vi "read_params.vi"(8 "error in (no error)":errorcluster, 11 "MLPRegressor in":refnum<class "MLPRegressor.lvclass">) -> (0 "error out":errorcluster, 2 "params":T1={"hidden_layer_sizes"=[100.0], "activation"="relu", "solver"="adam", "alpha"=0.0001, "batch_size"={"batch_size_type"="auto", "batch_size_int"=32.0}, "learning_rate"="constant", "learning_rate_init"=0.001, "power_t"=0.5, "max_iter"=200.0, "shuffle"=TRUE, "random_state"=0.0, "tol"=0.0001, "verbose"=FALSE, "warm_start"=FALSE, "momentum"=0.9, "nesterovs_momentum"=FALSE, "early_stopping"=FALSE, "validation_fraction"=0.1, "beta_1"=0.999, "beta_2"=0.999, "epsilon"=1e-08, "n_iter_no_change"=10.0, "max_fun"=15000.0}, 3 "MLPRegressor out":refnum<class "MLPRegressor.lvclass">)   [LabVIEW 2020, in "MLPRegressor.lvclass"]
uses:
  MLPRegressor.lvclass
  Controls/mlp_regressor_params.ctl
  MLPRegressor.lvclass/MLPRegressor.ctl
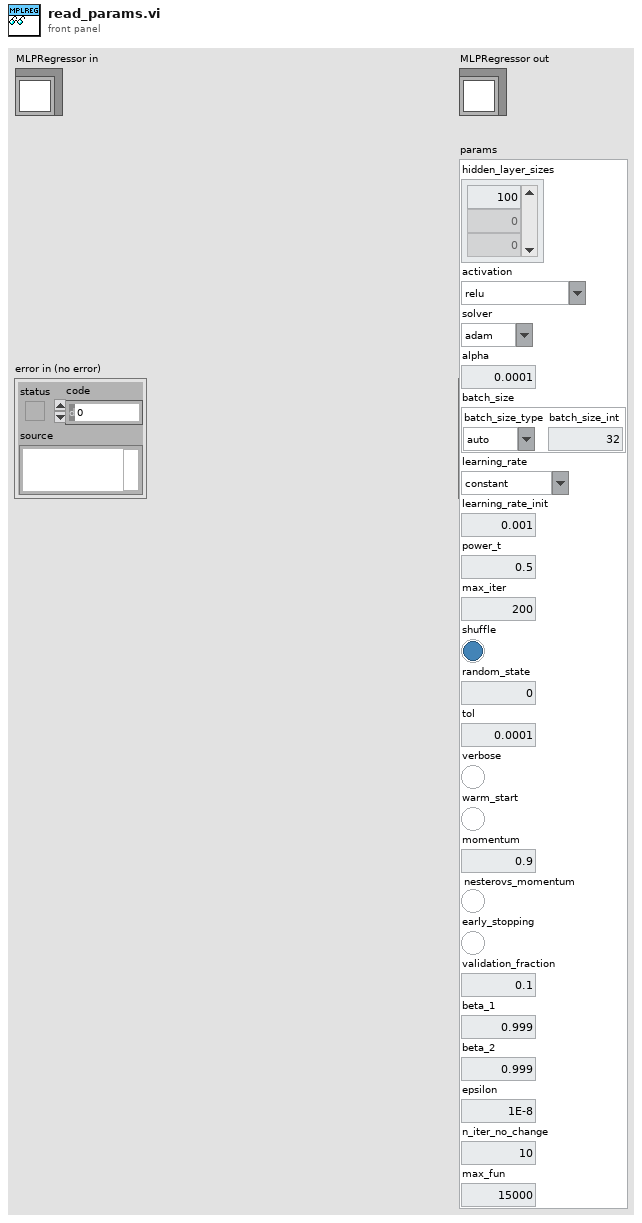
[diagram p1: front panel]
types:
  T1 = typedef "mlp_regressor_params.ctl" = cluster{"hidden_layer_sizes":dbl[], "activation":string, "solver":string, "alpha":dbl, "batch_size":cluster{"batch_size_type":string, "batch_size_int":dbl}, "learning_rate":string, "learning_rate_init":dbl, "power_t":dbl, "max_iter":dbl, "shuffle":bool, "random_state":dbl, "tol":dbl, "verbose":bool, "warm_start":bool, "momentum":dbl, "nesterovs_momentum":bool, "early_stopping":bool, "validation_fraction":dbl, "beta_1":dbl, "beta_2":dbl, "epsilon":dbl, "n_iter_no_change":dbl, "max_fun":dbl}
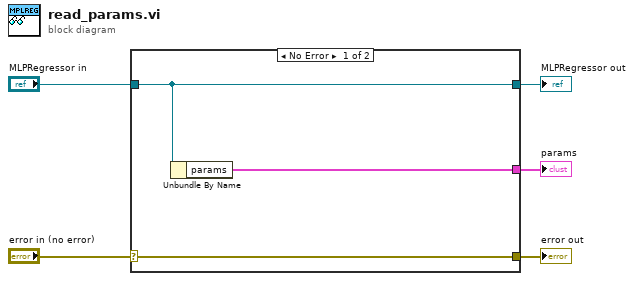
[diagram p0: block diagram]
diagram:
  n1 = case shown="No Error" "error in (no error)" {
    selector: "error in (no error)" -> [w8 w9]
    tunnel: [w8 w9] -> w4
    tunnel: [w7 w10] -> w2
    tunnel: "MLPRegressor in" -> [w7 w10]
    tunnel: [w6 _] -> w1
    frame No Error {
      n2 = Unbundle By Name(w7) -> ("params"=w6:T1)
    }
    frame Error {
    }
  }
  "error out" <- w4
  "MLPRegressor out" <- w2
  "params" <- w1
